vi "test------Execute Change Boolean Image.vi"(6 "Mouse Position":T1, 8 "User VI Ref":refnum<vi>, 9 "Menu Item Tag Suffix":string, 10 "Remaining Items":refnum<vi>[](array[refnum]), 11 "Affected Items":T2) -> (0 "Fail transaction?":bool)   [LabVIEW 2021]
doc: "This VI will set a Boolean type that is input to the control's tag and stays persistent. It marks the data that is used in future application when changing themes.\n\n<b>Original</b>:This VI is part of a plug-in for modifying the LabVIEW shortcut menus. This is the execute VI which is called when the shortcut menu is chosen by the user. It performs the action of the selected menu item."
uses:
  Set Boolean Type.llb/Set Boolean Type.ctl
  <vilib>/Utility/miscctls.llb/LVPositionTypeDef.ctl
panel:
  out "error out":errorcluster
  # "All controls on this panel except \"Affected Items\" have been locked to prevent accidental edits. Changing the control names or types, other than the elements of the \"Affected Items\" cluster will make the VI unusable as a menu plugin.\n\nSee Context Help for each control for details about its use."
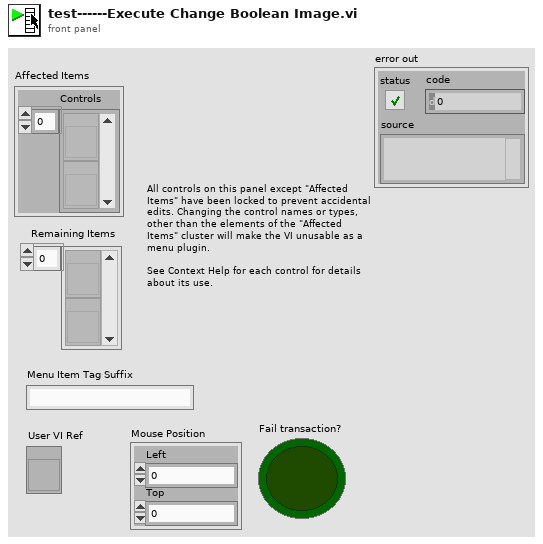
[diagram p1: front panel]
types:
  T1 = typedef "LVPositionTypeDef.ctl" = cluster{"Left":i32, "Top":i32}
  T2 = typedef "Set Boolean Type.ctl" = cluster{"Controls":refnum<vi>[]}
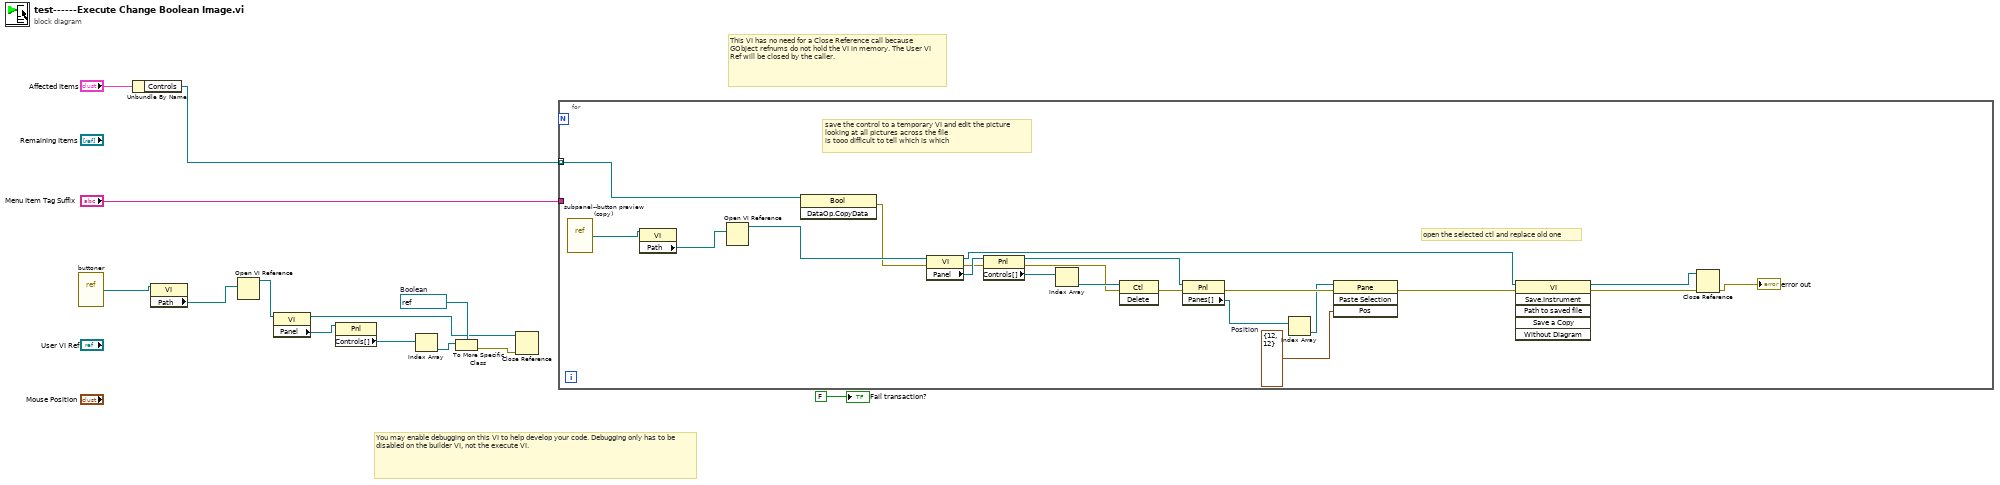
[diagram p0: block diagram]
diagram:
  w4 = refnum<vi> refnum  # Boolean
  # "You may enable debugging on this VI to help develop your code. Debugging only has to be disabled on the builder VI, not the execute VI."
  # "This VI has no need for a Close Reference call because GObject refnums do not hold the VI in memory. The User VI Ref will be closed by the caller."
  n1 = vi-ref "buttoner.vi"() -> (w9:refnum<vi>)
  n2 = Unbundle By Name("Affected Items") -> ("Controls"=w1:refnum<vi>[])
  n3 = property class="VI"(reference=w9) -> ("Path"=w10:path)  [unwired: 1 in, 2 out]
  n4 = Open VI Reference(vi path=w10) -> (vi reference=w8:refnum<vi>)  [unwired: 5 in, 1 out]
  n5 = property class="VI"(reference=w8) -> (reference out=w3:refnum<vi>, "Panel"=w7:refnum<vi>)  [unwired: 1 in, 1 out]
  n6 = property class="Pnl"(reference=w7) -> ("Controls[]"=w6:refnum<vi>[])  [unwired: 1 in, 2 out]
  n7 = Index Array(array=w6) -> (element=w5:refnum<vi>)  [unwired: 1 in]
  n8 = To More Specific Class(target class=w4, reference=w5) -> (error out=w2:errorcluster)  [unwired: 1 in, 1 out]
  n9 = Close Reference(reference=w3, error in (no error)=w2) -> ()  [unwired: 1 out]
  n10 = for {
    tunnel: w1 -> [w25] mode=indexing
    tunnel: "Menu Item Tag Suffix" -> [_]
    w14 = T1 {"Left"=12, "Top"=12}  # Position
    # "open the selected ctl and replace old one"
    # "save the control to a temporary VI and edit the picture\nlooking at all pictures across the file\nis tooo difficult to tell which is which"
    n11 = vi-ref "subpanel--button preview (copy).vi"() -> (w34:refnum<vi>)
    n12 = property class="VI"(reference=w34) -> ("Path"=w22:path)  [unwired: 1 in, 2 out]
    n13 = Open VI Reference(vi path=w22) -> (vi reference=w26:refnum<vi>)  [unwired: 5 in, 1 out]
    n14 = invoke class="Bool" method="DataOp.CopyData"(reference=w25) -> (error out=w24:errorcluster)  [unwired: 2 in, 2 out]
    n15 = property class="VI"(reference=w26, error in=w24) -> (reference out=w20:refnum<vi>, error out=w29:errorcluster, "Panel"=w33:refnum<vi>)
    n16 = property class="Pnl"(reference=w33, error in=w29) -> (reference out=w18:refnum<vi>, error out=w28:errorcluster, "Controls[]"=w32:refnum<vi>[])
    n17 = Index Array(array=w32) -> (element=w31:refnum<vi>)  [unwired: 1 in]
    n18 = invoke class="Ctl" method="Delete"(reference=w31, error in=w28) -> (error out=w30:errorcluster)  [unwired: 1 in, 2 out]
    n19 = property class="Pnl"(reference=w18, error in=w30) -> (error out=w19:errorcluster, "Panes[]"=w17:refnum<vi>[])  [unwired: 1 out]
    n20 = Index Array(array=w17) -> (element=w16:refnum<vi>)  [unwired: 1 in]
    n21 = invoke class="Pane" method="Paste Selection"(reference=w16, error in=w19, "Pos"=w14) -> (error out=w21:errorcluster)  [unwired: 1 in, 3 out]
    n22 = invoke class="VI" method="Save.Instrument"(reference=w20, error in=w21) -> (reference out=w23:refnum<vi>, error out=w27:errorcluster)  [unwired: 4 in, 4 out]
    n23 = Close Reference(reference=w23, error in (no error)=w27) -> (error out=→"error out":errorcluster)
  }
  "Fail transaction?" <- FALSE ("Fail transaction?")
